vi "TI Sensored BLDC (RT).vi"() -> ()   [LabVIEW 2013]
uses:
  <vilib>/rvi/interface/nirviOpenFPGA/nirviOpenFPGA.xnode
  <vilib>/rvi/interface/nirviReadWriteControl/nirviReadWriteControl.xnode
  <vilib>/rvi/interface/Simulation/niFpgaSimulationCallBeginRW.vi
  <vilib>/rvi/errors/niLvFpgaAdjustHostInterfaceError.vi
  NiFpgaLv.dll
  <vilib>/Utility/error.llb/Error Cluster From Error Code.vi
  FPGA Bitfiles/TIsbRIO_FPGATarget_TISensoredBLDC(F_DyXSZt47tvg.lvbitx
  FPGA/TI Sensored BLDC (FPGA).vi
  <vilib>/FPGAPlugInAG/sbRIO-9626/niLvFpga_Open_sbRIO-9626.vi
  <vilib>/rvi/interface/common/dynamic/niFpgaDynamicAddResources.vi
panel:
  out "error out":errorcluster
  out "Position (Counts)":i32
  in  "PWM Enable":bool
  in  "Zero Position":bool
  in  "Align Rotor":bool
  out "Rotor Position (deg)":dbl=43.25
  in  "Phase Advance (deg)":dbl=3.0 format="%.2f"
  in  "Phases (deg)":dbl[](array[numeric])=[0.0, 30.0, 60.0, 90.0, 120.0, 150.0, 180.0, 210.0, 240.0, 270.0, 300.0, 330.0, 360.0] format="%.2f"
  in  "Duty (%)":dbl=50.0 format="%.2f"
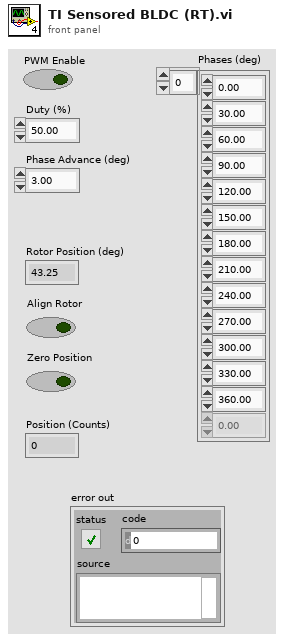
[diagram p1: front panel]
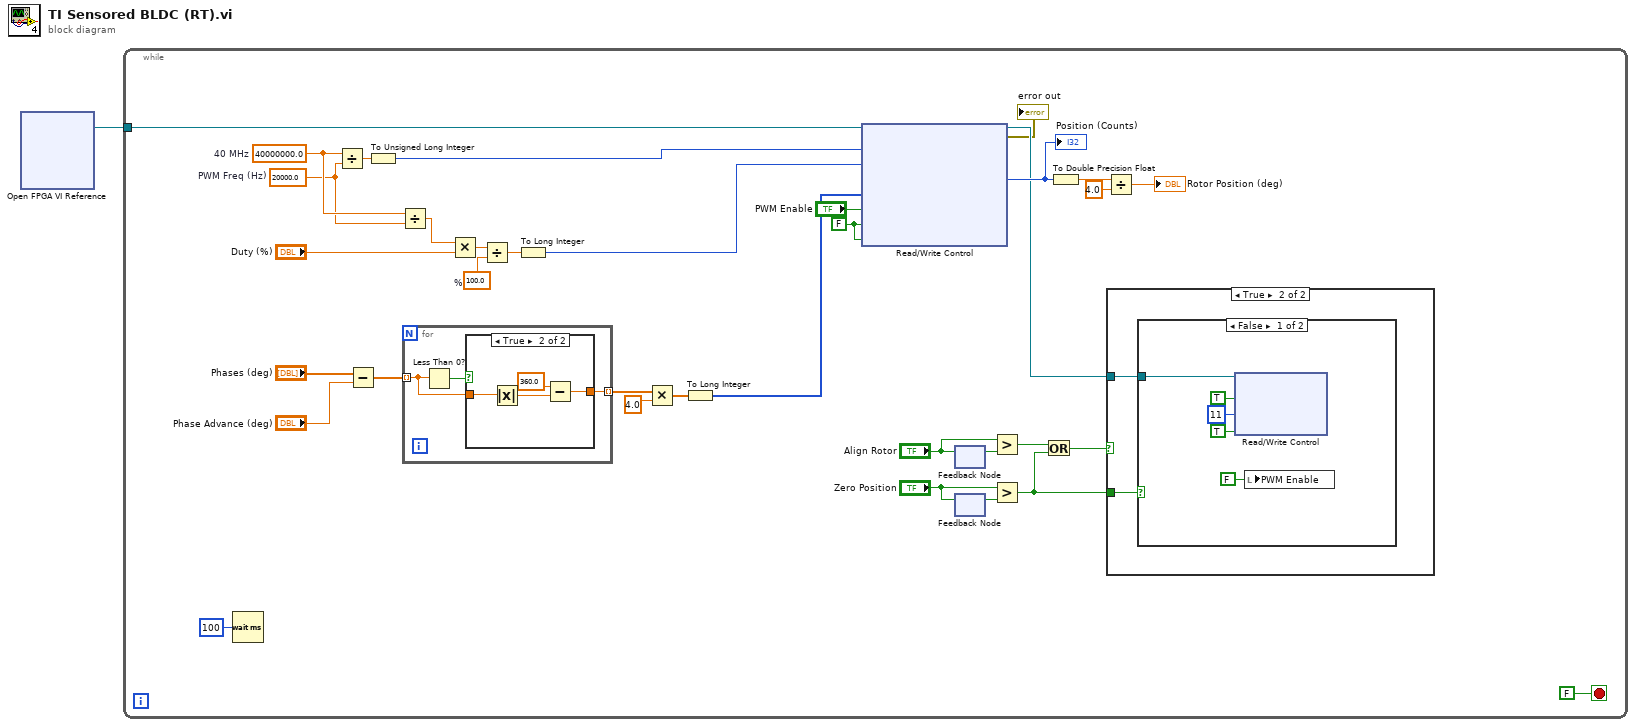
[diagram p0: block diagram]
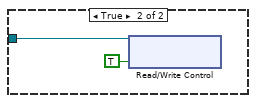
[diagram p3: hidden frame]
diagram:
  n1 = xnode "Open FPGA VI Reference"() -> ("FPGA VI Reference Out"=w1:refnum<k20>)  [unwired: 2 in, 1 out]
  n2 = while {
    tunnel: w1 -> [w35]
    stop <- FALSE stop-if-true
    w3 = FALSE ("Manual")
    w32 = 20000.0  # PWM Freq (Hz)
    w34 = 40000000.0  # 40 MHz
    w29 = 100.0  # %
    n3 = Wait (ms)(milliseconds to wait=u32 100) -> ()  [unwired: 1 out]
    n4 = Divide(x=w34, y=w32) -> (x/y=w31:dbl)
    n5 = Subtract(x="Phases (deg)", y="Phase Advance (deg)") -> (x-y=w18:dbl[])
    n6 = To Unsigned Long Integer(number=w31) -> (unsigned 32bit integer=w26:u32)
    n7 = Divide(x=w34, y=w32) -> (x/y=w27:dbl)
    n8 = for {
      tunnel: w18 -> [w47] mode=indexing
      tunnel: [w46] -> w16 mode=indexing
      n9 = Less Than 0?(x=w47) -> (x < 0?=w48:bool)
      n10 = case shown="True" w48 {
        tunnel: w47 -> [w49 w53]
        tunnel: [w49 w50] -> w46
        frame False {
        }
        frame True {
          n11 = Absolute Value(x=w53) -> (abs(x)=w52:dbl)
          n12 = Subtract(x=360.0, y=w52) -> (x-y=w50:dbl)
        }
      }
    }
    n13 = Multiply(x=w27, y="Duty (%)") -> (x*y=w30:dbl)
    n14 = Divide(x=w30, y=w29) -> (x/y=w28:dbl)
    n15 = To Long Integer(number=w28) -> (32bit integer=w25:i32)
    n16 = Multiply(x=w16, y=4.0) -> (x*y=w14:dbl[])
    n17 = To Long Integer(number=w14) -> (32bit integer=w13:i32[])
    n18 = xnode "Read/Write Control"("FPGA VI Reference In"=w35, "PWM Period (Ticks)"=w26, "PWM Duty Cycle (Ticks)"=w25, "Phase Positions"=w13, "PWM Enable"="PWM Enable", "Manual"=w3, "Position Reset"=w3) -> ("FPGA VI Reference Out"=w4:refnum<k20>, "error out"=→"error out":errorcluster, "Position (Counts)"=w24:i32)  [unwired: 1 in]
    "Position (Counts)" <- w24
    n19 = feedback-in #1("Align Rotor") -> ()
    n20 = feedback #1() -> (w11:bool)  [unwired: 1 in]
    n21 = feedback #2() -> (w10:bool)  [unwired: 1 in]
    n22 = feedback-in #2("Zero Position") -> ()
    n23 = Greater?(x="Align Rotor", y=w11) -> (0:w8:bool)
    n24 = Greater?(x="Zero Position", y=w10) -> (0:w6:bool)
    n25 = Or(x=w8, y=w6) -> (x .or. y?=w7:bool)
    n26 = To Double Precision Float(number=w24) -> (double precision float=w23:dbl)
    n27 = Divide(x=w23, y=4.0) -> (x/y=→"Rotor Position (deg)":dbl)
    n28 = case shown="True" w7 {
      tunnel: w6 -> [_ w38]
      tunnel: w4 -> [_ w37]
      frame False {
      }
      frame True {
        n29 = case shown="False" w38 {
          tunnel: w37 -> [w41 w45]
          frame False {
            n30 = xnode "Read/Write Control"("FPGA VI Reference In"=w41, "Manual"=TRUE ("PWM Enable"), "Manual Phase"=u8 11, "PWM Enable"=TRUE ("Align")) -> ()  [unwired: 1 in, 2 out]
            n31 = local write "PWM Enable"(FALSE ("PWM Enable")) -> ()
          }
          frame True {
            n32 = xnode "Read/Write Control"("FPGA VI Reference In"=w45, "Position Reset"=TRUE) -> ()  [unwired: 1 in, 2 out]
          }
        }
      }
    }
  }
